vi "Join Byte.vi"() -> ()   [LabVIEW 2021]
panel:
  in  "LSB Length":u8=4
  in  "LSB":u8 format="%x"
  in  "MSB":u8 format="%x"
  out "Byte":u8 format="%x"
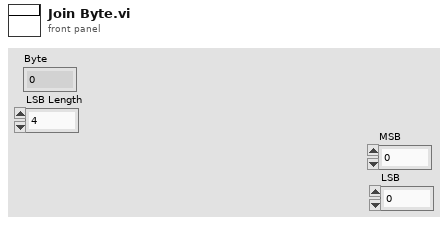
[diagram p1: front panel]
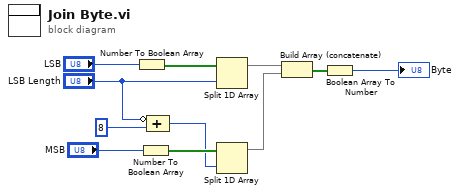
[diagram p0: block diagram]
diagram:
  n1 = Number To Boolean Array(number="LSB") -> (Boolean array=w8:bool[])
  n2 = Number To Boolean Array(number="MSB") -> (Boolean array=w7:bool[])
  n3 = Compound Arithmetic op=ADD(invert "LSB Length", u8 8 ("value")) -> (w6:u8)
  n4 = Split 1D Array(array=w8, index="LSB Length") -> (first subarray=w5:bool[])  [unwired: 1 out]
  n5 = Split 1D Array(array=w7, index=w6) -> (first subarray=w4:bool[])  [unwired: 1 out]
  n6 = Build Array (concatenate)(w5, w4) -> (w3:bool[])
  n7 = Boolean Array To Number(Boolean array=w3) -> (number=→"Byte":u8)
